vi "Destroy.vi"(8 "error in (no error)":errorcluster, 11 "TopLevel in":refnum<class "GIS Printer.lvclass">) -> (0 "error out":errorcluster, 3 "TopLevel out":refnum<class "GIS Printer.lvclass">)   [LabVIEW 2022 SP3, in "GIS Printer.lvclass"]
uses:
  GIS Printer.lvclass
  GIS Printer.lvclass/GIS Printer.ctl
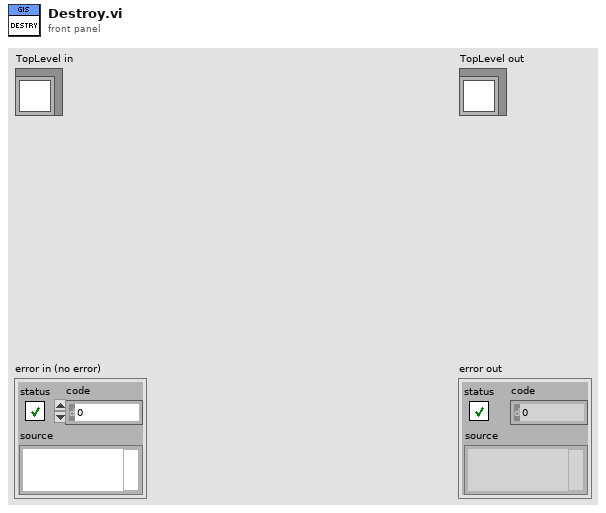
[diagram p1: front panel]
types:
  T1 = typedef "GIS Printer.lvclass/Private Data.ctl" = cluster{"UserEvents":T2, "All Dependencies":cluster{"Class References":refnum<class>[], "Class Names":string[]}, "PrinterConiguration":T3, "Status":T4, "GISHeadStatus":T5[], "HeadStatus":T6}
  T2 = typedef "GIS Printer.lvclass/UserEvents.ctl" = cluster{"API Incoming Event":refnum<user-event>, "API Executed Event":refnum<user-event>, "API Return Event":refnum<user-event>, "Status Changed Event":refnum<user-event>, "Abort":refnum<user-event>, "stop process":refnum<user-event>, "GISPollStatus":refnum<user-event>, "GISHeadStatus":refnum<user-event>, "Error Event":refnum<user-event>}
  T3 = typedef "GIS Printer.lvclass/PrinterConfiguration--Cluster.ctl" = cluster{"IPAddress":string, "Move Stage on RTP Command?":bool, "Stage Move Position":string, "PH1-Prime Path":path, "PH2-Prime Path":path, "PH3-Prime Path":path, "PH4-Prime Path":path, "PH5-Prime Path":path, "PH6-Prime Path":path, "PrintScriptsFolder":path, "PurgeScriptsFolder":path, "StageScriptsFolder":path, "PH1-HeatOn Path":path, "PH2-HeatOn Path":path, "PH3-HeatOn Path":path, "PH4-HeatOn Path":path, "PH5-HeatOn Path":path, "PH6-HeatOn Path":path, "PH1-HeatOff Path":path, "PH2-HeatOff Path":path, "PH3-HeatOff Path":path, "PH4-HeatOff Path":path, "PH5-HeatOff Path":path, "PH6-HeatOff Path":path}
  T4 = typedef "GIS Printer.lvclass/Status Cluster.ctl" = cluster{"Command Status":variant, "TCP Commands & Responses":string[][], "Printer Busy?":bool}
  T5 = typedef "GIS Status--Cluster.ctl" = cluster{"HeadEnabled":bool, "SpitEnabled":bool, "HeaterEnabled":bool, "TargetTemperature":dbl, "CurrentTemperature":dbl}
  T6 = typedef "HeadEnableStatus--cluster.ctl" = cluster{"PH1_Enable":bool, "PH2_Enable":bool, "PH3_Enable":bool, "PH4_Enable":bool, "PH5_Enable":bool, "PH6_Enable":bool}
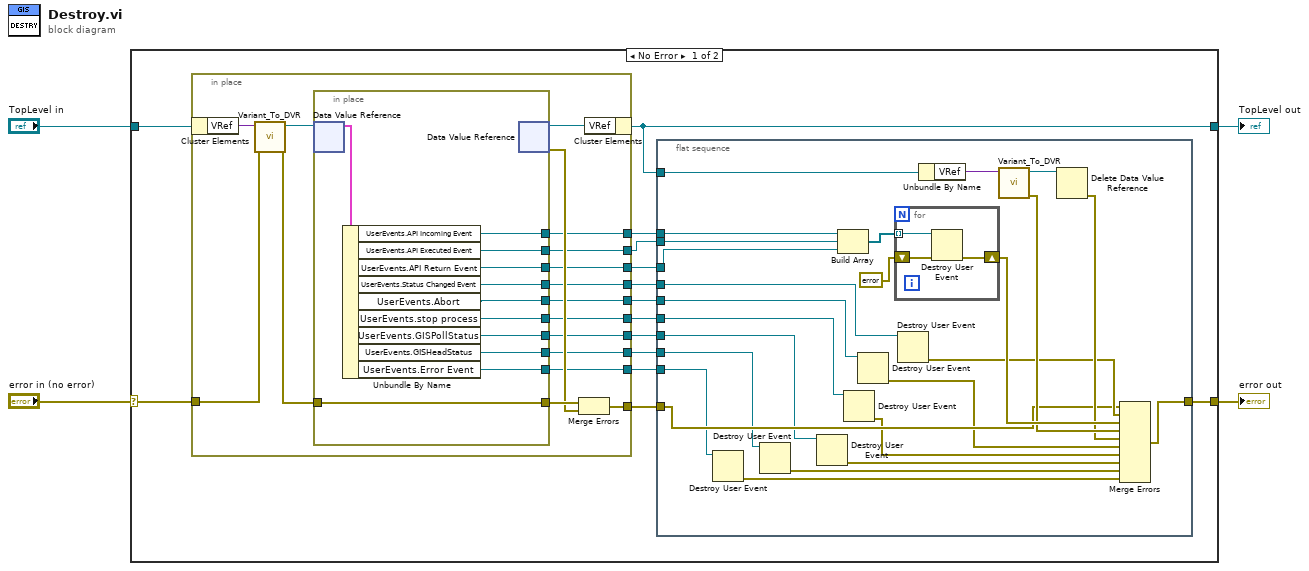
[diagram p0: block diagram]
diagram:
  n1 = case shown="No Error" "error in (no error)" {
    selector: "error in (no error)" -> [w17 w76]
    tunnel: [w13 w76] -> w3
    tunnel: [w14 w75] -> w1
    tunnel: "TopLevel in" -> [w18 w75]
    frame No Error {
      n2 = in-place {
        in-place-border: w17 -> [w60]
        in-place-border: [w56] -> w15
        in-place-border: [w55] -> w16
        in-place-border: [w54] -> w12
        in-place-border: [w53] -> w11
        in-place-border: [w52] -> w10
        in-place-border: [w51] -> w9
        in-place-border: [w50] -> w8
        in-place-border: [w49] -> w7
        in-place-border: [w48] -> w6
        in-place-border: [w47] -> w5
        n3 = in-place-cluster #1(w18) -> ("VRef"=w63:variant)
        n4 = call "Variant_To_DVR.vi"("error in (no error)"=w60, "Variant"=w63) -> ("error out"=w59:errorcluster, "DVR"=w62:refnum<data-value>)  [unwired: 8 in]
        n5 = in-place {
          in-place-border: [w73] -> w55
          in-place-border: w59 -> [w72]
          in-place-border: [w72] -> w58
          in-place-border: [w71] -> w54
          in-place-border: [w70] -> w53
          in-place-border: [w69] -> w52
          in-place-border: [w68] -> w51
          in-place-border: [w67] -> w50
          in-place-border: [w66] -> w49
          in-place-border: [w65] -> w48
          in-place-border: [w64] -> w47
          n6 = in-place-dvr #2(w62) -> (w74:T1)  [unwired: 1 out]
          n7 = Unbundle By Name(w74) -> ("UserEvents.API Incoming Event"=w73:refnum<user-event>, "UserEvents.API Executed Event"=w71:refnum<user-event>, "UserEvents.API Return Event"=w70:refnum<user-event>, "UserEvents.Status Changed Event"=w69:refnum<user-event>, "UserEvents.Abort"=w68:refnum<user-event>, "UserEvents.stop process"=w67:refnum<user-event>, "UserEvents.GISPollStatus"=w66:refnum<user-event>, "UserEvents.GISHeadStatus"=w65:refnum<user-event>, "UserEvents.Error Event"=w64:refnum<user-event>)
          n8 = in-place-dvr #2() -> (w61:refnum<data-value>, w57:errorcluster)  [unwired: 1 in]
        }
        n9 = Merge Errors(w58, w57) -> (w56:errorcluster)
        n10 = in-place-cluster #1("VRef"=w61) -> (w14:refnum<class "GIS Printer.lvclass">)
      }
      n11 = flat-sequence {
        tunnel: w16 -> [w43]
        tunnel: w15 -> [w29]
        tunnel: w14 -> [w40]
        tunnel: [w36] -> w13
        tunnel: w12 -> [w33]
        tunnel: w11 -> [w32]
        tunnel: w10 -> [w31]
        tunnel: w9 -> [w28]
        tunnel: w8 -> [w27]
        tunnel: w7 -> [w24]
        tunnel: w6 -> [w22]
        tunnel: w5 -> [w20]
        frame #0 {
          n12 = Destroy User Event(user event=w20) -> (error out=w19:errorcluster)  [unwired: 1 in]
          n13 = Destroy User Event(user event=w22) -> (error out=w21:errorcluster)  [unwired: 1 in]
          n14 = Destroy User Event(user event=w24) -> (error out=w23:errorcluster)  [unwired: 1 in]
          n15 = Build Array(w43, w33, w32) -> (w42:refnum<user-event>[])
          n16 = Destroy User Event(user event=w27) -> (error out=w25:errorcluster)  [unwired: 1 in]
          n17 = Destroy User Event(user event=w28) -> (error out=w26:errorcluster)  [unwired: 1 in]
          n18 = for {
            tunnel: w42 -> [w46] mode=indexing
            shift-right: [w45] -> w37
            shift-left: errorcluster {"status"=FALSE, "code"=0, "source"=""} ("error constant") -> [w44]
            n19 = Destroy User Event(user event=w46, error in=w44) -> (error out=w45:errorcluster)
          }
          n20 = Destroy User Event(user event=w31) -> (error out=w30:errorcluster)  [unwired: 1 in]
          n21 = Unbundle By Name(w40) -> ("VRef"=w39:variant)
          n22 = call "Variant_To_DVR.vi"("Variant"=w39) -> ("error out"=w35:errorcluster, "DVR"=w38:refnum<data-value>)  [unwired: 9 in]
          n23 = Delete Data Value Reference(data value reference=w38) -> (error out=w34:errorcluster)  [unwired: 1 in, 1 out]
          n24 = Merge Errors(w29, w30, w37, w35, w34, w26, w25, w23, w21, w19) -> (w36:errorcluster)
        }
      }
    }
    frame Error {
    }
  }
  "error out" <- w3
  "TopLevel out" <- w1
